vi "RegisteredMessages.vi"() -> (3 "registered messages":string[](array[string]))   [LabVIEW 2017, in "TrendAlarm.lvlib"]
uses:
  <vilib>/addons/InsightCM/Devices/Shared/Common/TrendAlarm/TrendAlarm.lvlib
  <vilib>/addons/InsightCM/Devices/Shared/Common/ServerComm/ServerComm.lvlib
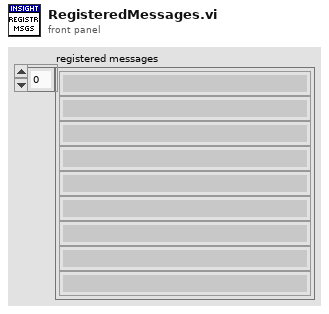
[diagram p1: front panel]
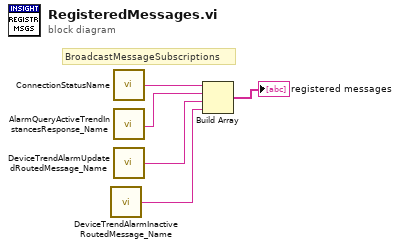
[diagram p0: block diagram]
diagram:
  # "BroadcastMessageSubscriptions"
  n1 = call <vilib>:"DeviceTrendAlarmInactiveRoutedMessage_Name.vi"() -> ("MessageName"=w1:string)  [unwired: 5 in]
  n2 = call <vilib>:"ConnectionStatusName.vi"() -> ("message name"=w5:string)  [unwired: 5 in]
  n3 = call <vilib>:"AlarmQueryActiveTrendInstancesResponse_Name.vi"() -> ("MessageName"=w2:string)  [unwired: 5 in]
  n4 = call <vilib>:"DeviceTrendAlarmUpdatedRoutedMessage_Name.vi"() -> ("MessageName"=w3:string)  [unwired: 5 in]
  n5 = Build Array(w5, w2, w3, w1) -> (→"registered messages":string[])
